vi "NearFiledCamConnect.vi"(2 "错误输入（无错误）":errorcluster) -> (0 "错误输出":errorcluster, 1 "连接状态":bool)   [LabVIEW 2018]
panel:
  out "采集套接字":i32
  out "控制套接字":i32
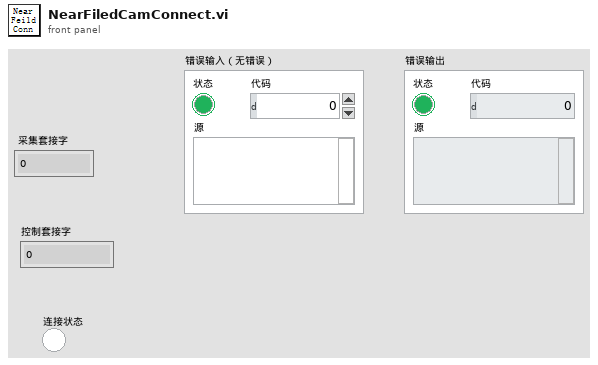
[diagram p1: front panel]
types:
  T1 = typedef "Image Type" = u32
  T2 = typedef "IMAQ Image.ctl" = refnum<image>
  T3 = cluster{"示波器":cluster{"Channel (0:Channel 1)":enum16{"Channel 1", "Channel 2", "Channel 3", "Channel 4"}, "电压范围":dbl, "触发电压":dbl, "时间范围":dbl, " 示波器VISA":refnum<visa-resource-name>, "时间范围 标签":u64, "电压范围 标签":u64, "触发电压 标签":u64, "输入阻抗/Ω":u64}, "光谱仪":cluster{"SpecDataReference":refnum<queue>, "grating center":dbl, "Exposure Time (s)":dbl, "是否进行详细设置":bool, " 开始通信检查":bool, "通信成功？":bool, "波长":dbl}, " 近场相机":cluster{"曝光时间/100us":dbl, "模拟增益":i32, "控制套接字":i32, "IP 地址":string, " 采集套接字":i32, "  版本号":i32, "ImageData":T2, "  增益最大":i32, "  增益最小":i32, " 曝光最大":i32, " 曝光最小":i32, " 帧速":i32, " 同步切换":i32, "  曝光缩放":i32}, " 偏振仪":cluster{"电压范围":u64, "触发电压":u64, "时间范围":u64, "波长范围":enum16{"可见光 400-700nm", "近红外 700-1100nm"}, "可见光偏振测量仪VISA":refnum<visa-resource-name>, "近红外偏振测量仪VISA":refnum<visa-resource-name>}, " 功率计":cluster{"通道":enum16{"Channel 1", "Channel 2"}, "工作波长":u32, "单位":u64, "时间范围":u64, "IP地址":string, "端口":u32}, "能量计":cluster{"通道":enum16{"Channel 1", "Channel 2"}, "工作波长":u32, "单位":u64, "时间范围":u64, "IP地址":string, "端口":u32, "能量计量程":enum16{"200uJ", "20uJ", "2uJ", "200nJ"}}, "电机":cluster{"Channel (0:Channel 1)":enum16{"Channel 1", "Channel 2", "Channel 3", "Channel 4"}, "电压范围":u64, "触发电压":u64, "时间范围":u64}, " 远场相机":cluster{"曝光时间":i32, "模拟增益":i32, "控制套接字":i32, "IP 地址":string, " 采集套接字":i32, "  版本号":i32, "ImageData":T2, "  增益最大":i32, "  增益最小":i32, " 曝光最大":i32, " 曝光最小":i32, " 帧速":i32, " 同步切换":i32, "  曝光缩放":i32, "ImageData B":T2}}
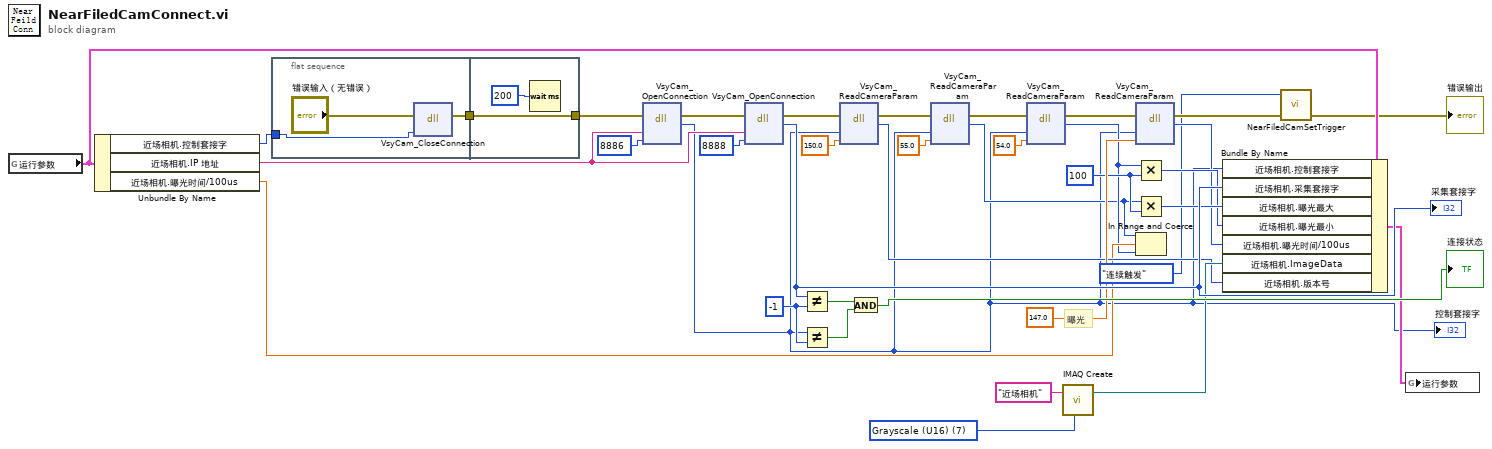
[diagram p0: block diagram]
diagram:
  w14 = 100 ("y")
  w21 = T1 7 items=["Grayscale (U8)", "Grayscale (I16)", "Grayscale (SGL)", "Complex (CSG)", "RGB (U32)", "HSL (U32)", "RGB (U64)", "Grayscale (U16)"] ("Image Type")
  w33 = -1
  # "曝光"
  n1 = global read "参数.vi" "运行参数"() -> (w29:T3)
  n2 = Unbundle By Name(w29) -> ("近场相机.控制套接字"=w5:i32, "近场相机.IP 地址"=w34:string, "近场相机.曝光时间/100us"=w11:dbl)
  n3 = flat-sequence {
    tunnel: [w40] -> w8
    tunnel: w5 -> [w38]
    tunnel: [w42] -> w15
    tunnel: w8 -> [w42]
    frame #0 {
      n4 = dll-call lib="PTH2^abs E航天测量驱动相机驱动LabView2014Demo_V1.0.8\nLabView14Demo\nVsyCam.dll" fn="VsyCam_CloseConnection"(error in="错误输入（无错误）", "sockFd"=w38) -> (error out=w40:errorcluster)  [unwired: 4 in, 1 out]
    }
    frame #1 {
      n5 = Wait (ms)(milliseconds to wait=u32 200 ("等待时间（毫秒）")) -> ()  [unwired: 1 out]
    }
  }
  n6 = dll-call lib="PTH2^abs E航天测量驱动相机驱动LabView2014Demo_V1.0.8\nLabView14Demo\nVsyCam.dll" fn="VsyCam_OpenConnection"(error in=w15, "ip"=w34, "port"=8886) -> (error out=w36:errorcluster, "返回类型"=w3:i32)  [unwired: 4 in, 1 out]
  "控制套接字" <- w3
  n7 = dll-call lib="PTH2^abs E航天测量驱动相机驱动LabView2014Demo_V1.0.8\nLabView14Demo\nVsyCam.dll" fn="VsyCam_OpenConnection"(error in=w36, "ip"=w34, "port"=8888) -> (error out=w18:errorcluster, "返回类型"=w28:i32)  [unwired: 4 in, 1 out]
  "采集套接字" <- w28
  n8 = Not Equal?(x=w28, y=w33) -> (x != y?=w32:bool)
  n9 = Not Equal?(x=w3, y=w33) -> (x != y?=w31:bool)
  n10 = dll-call lib="PTH2^abs E航天测量驱动相机驱动LabView2014Demo_V1.0.8\nLabView14Demo\nVsyCam.dll" fn="VsyCam_ReadCameraParam"(error in=w18, "sockFd"=w3, "cmd"=150.0) -> (error out=w17:errorcluster, "返回类型"=w16:i32)  [unwired: 4 in, 1 out]
  n11 = And(x=w32, y=w31) -> (x .and. y?=→"连接状态":bool)
  n12 = dll-call lib="PTH2^abs E航天测量驱动相机驱动LabView2014Demo_V1.0.8\nLabView14Demo\nVsyCam.dll" fn="VsyCam_ReadCameraParam"(error in=w17, "sockFd"=w3, "cmd"=55.0) -> (error out=w24:errorcluster, "返回类型"=w6:i32)  [unwired: 4 in, 1 out]
  n13 = dll-call lib="PTH2^abs E航天测量驱动相机驱动LabView2014Demo_V1.0.8\nLabView14Demo\nVsyCam.dll" fn="VsyCam_ReadCameraParam"(error in=w24, "sockFd"=w3, "cmd"=54.0) -> (error out=w7:errorcluster, "返回类型"=w9:i32)  [unwired: 4 in, 1 out]
  n14 = call "IMAQ Create"("Image Name"="近场相机", "Image Type"=w21) -> ("New Image"=w20:T2)  [unwired: 3 in, 1 out]
  n15 = dll-call lib="PTH2^abs E航天测量驱动相机驱动LabView2014Demo_V1.0.8\nLabView14Demo\nVsyCam.dll" fn="VsyCam_ReadCameraParam"(error in=w7, "sockFd"=w3, "cmd"=147.0) -> (error out=w4:errorcluster, "返回类型"=w10:i32)  [unwired: 4 in, 1 out]
  n16 = Multiply(x=w9, y=w14) -> (x*y=w12:i32)
  n17 = Multiply(x=w6, y=w14) -> (x*y=w13:i32)
  n18 = In Range and Coerce(upper limit=w6, x=w11, lower limit=w9) -> ()  [unwired: 2 out]
  n19 = Bundle By Name(cluster=w29, "近场相机.控制套接字"=w3, "近场相机.采集套接字"=w28, "近场相机.曝光最大"=w13, "近场相机.曝光最小"=w12, "近场相机.曝光时间/100us"=w10, "近场相机.ImageData"=w20, "近场相机.版本号"=w16) -> (w27:T3)
  n20 = call "NearFiledCamSetTrigger.vi"("错误输入（无错误）"=w4, "触发模式"=enum16{"连续触发", "外部触发1", "外部触发2"}."连续触发") -> ("错误输出"=→"错误输出":errorcluster)  [unwired: 3 in]
  n21 = global write "参数.vi" "运行参数"(w27) -> ()
